vi "Facade.vi"(0 "Data In":T7, 2 "Display State In":T5, 3 "Container State":T6) -> (6 "Data Out":T7, 7 "Display State Out":T5, 8 "Action":T4)   [LabVIEW 2020, in "Input Criteria Table.xctl"]
uses:
  Input Criteria Table.xctl
  Data.vi
  Digital Input VIs/Tosca-Input Criterion.ctl
  epl-vi-lib/Utility VIs/Type Defs/Logic State.ctl
  <vilib>/_xctls/Container State.ctl
  State.vi
  <vilib>/_xctls/Action.ctl
  Input Criterion/Input Criterion.xctl
  Input Criterion/Data.vi
  <vilib>/_xctls/XControlSupport.lvlib
panel:
  in  "Crit5":T3(xcontrol)
  in  "Crit4":T3(xcontrol)
  in  "Crit3":T3(xcontrol)
  in  "Crit2":T3(xcontrol)
  in  "Crit1":T3(xcontrol)
  in  "Crit0":T3(xcontrol)
types:
  T1 = typedef "Tosca-Input Criterion.ctl" = cluster{"DigInput":i32, "State":T2, "Time (ms)":i32, "Name":string}
  T2 = typedef "Logic State.ctl" = enum16{"Low", "High", "Rising", "Falling"}
  T3 = cluster{"Criterion":T1, "Operator":i16, "visible":bool}
  T4 = typedef "XControlSupport.lvlib/Action.ctl" = cluster{"Data Changed?":bool, "State Changed?":bool, "Action Name":string}
  T5 = typedef "Input Criteria Table.xctl/State.vi" = cluster{"DI":string[], "Flags":string[]}
  T6 = typedef "XControlSupport.lvlib/Container State.ctl" = cluster{"Indicator?":bool, "Run Mode?":bool, " Refnum":refnum<vi>}
  T7 = typedef "Input Criteria Table.xctl/Data.vi" = cluster{"Name":string, "Criteria":T1[], "Operators":enum16{"AND", "OR"}[]}
  T8 = typedef "Input Criterion.xctl/Data.vi" = cluster{"Criterion":T1, "Operator":i16, "visible":bool}
  T9 = cluster{"Criteria":T1, "Operator":i32, "Visible":bool}
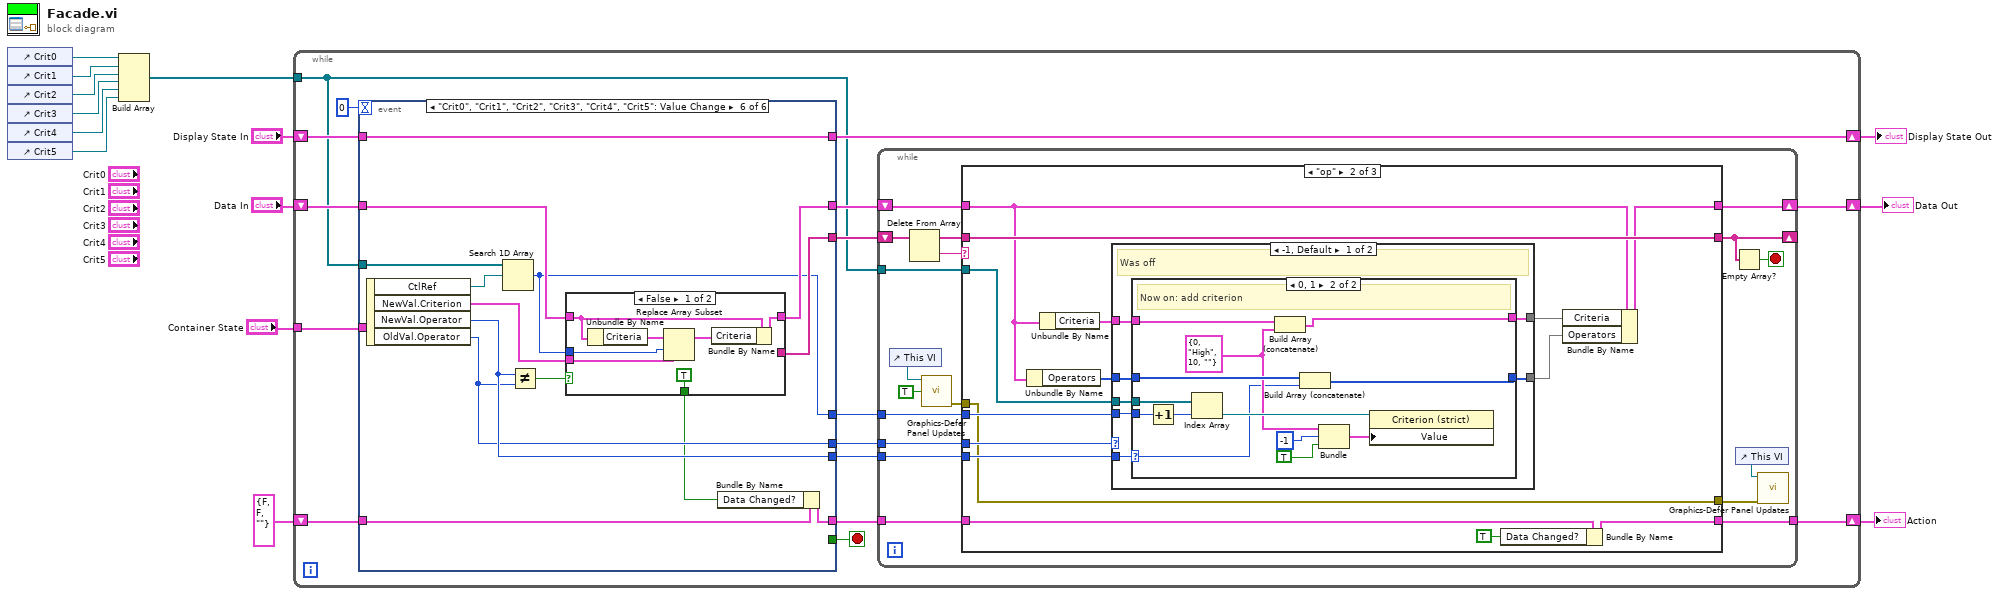
[diagram p0: block diagram]
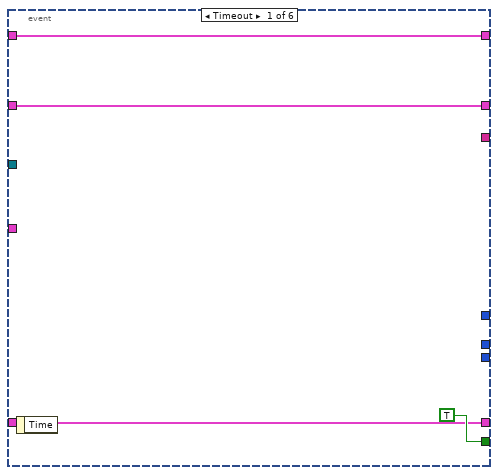
[diagram p2: hidden frame]
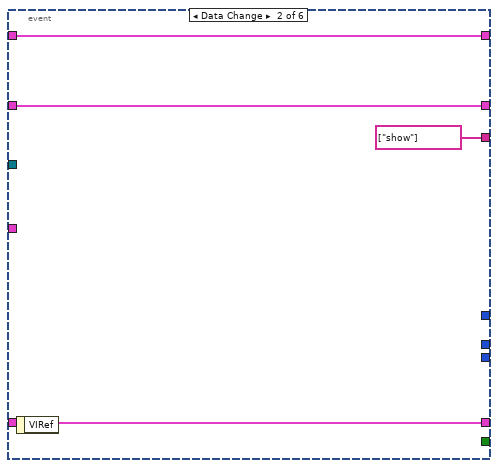
[diagram p3: hidden frame]
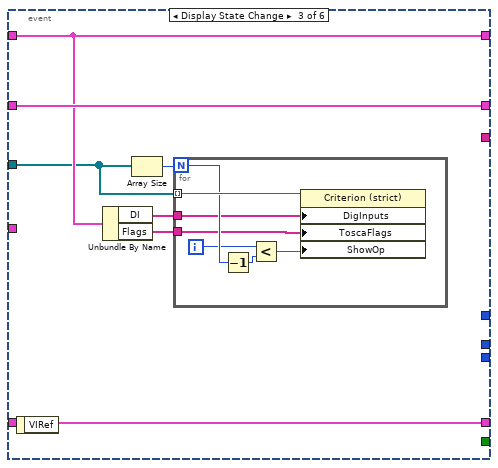
[diagram p4: hidden frame]
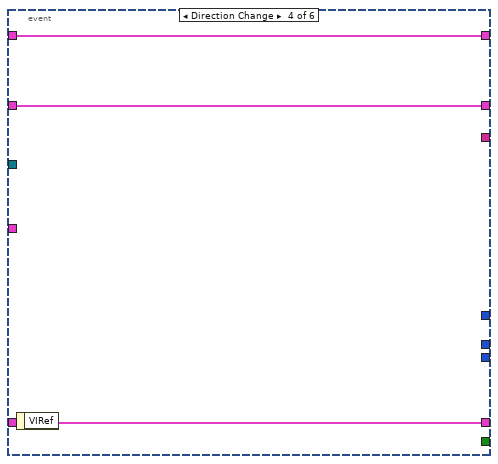
[diagram p5: hidden frame]
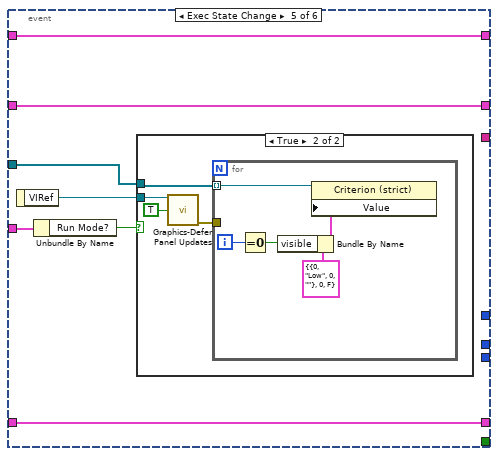
[diagram p6: hidden frame]
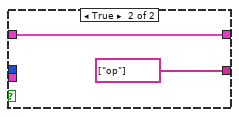
[diagram p8: hidden frame]
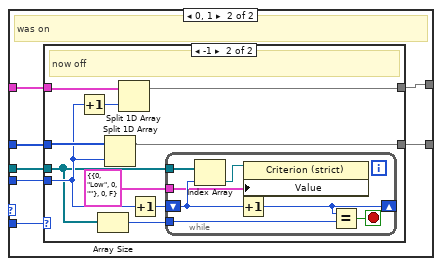
[diagram p11: hidden frame]
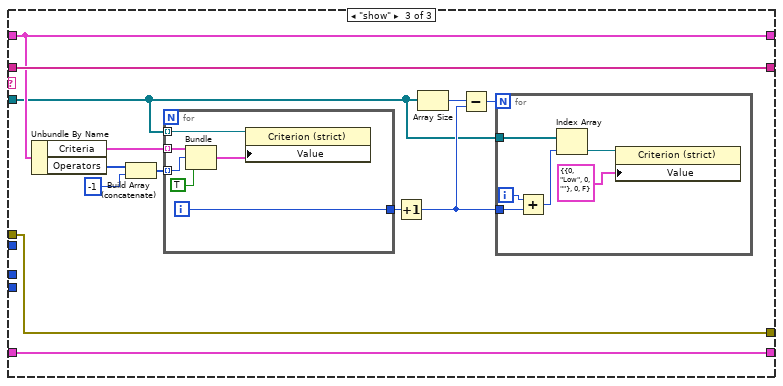
[diagram p13: hidden frame]
diagram:
  n1 = control-ref of="Crit0"() -> (w7:refnum<vi>)
  n2 = control-ref of="Crit1"() -> (w6:refnum<vi>)
  n3 = control-ref of="Crit2"() -> (w5:refnum<vi>)
  n4 = control-ref of="Crit3"() -> (w4:refnum<vi>)
  n5 = control-ref of="Crit4"() -> (w3:refnum<vi>)
  n6 = control-ref of="Crit5"() -> (w2:refnum<vi>)
  n7 = Build Array(w7, w6, w5, w4, w3, w2) -> (w1:refnum<vi>[])
  n8 = while {
    shift-right: [w29] -> w11
    shift-left: "Display State In" -> [w30]
    tunnel: "Container State" -> [w26]
    shift-right: [w18] -> w14
    shift-left: "Data In" -> [w25]
    shift-right: [w20] -> w9
    shift-left: T4 {"Data Changed?"=FALSE, "State Changed?"=FALSE, "Action Name"=""} ("Action") -> [w24]
    tunnel: w1 -> [w16]
    stop <- w28 stop-if-true
    n9 = event shown="[5] \"Crit0\", \"Crit1\", \"Crit2\", \"Crit3\", \"Crit4\", \"Crit5\": Value Change" {
      selector: _ -> [_ _ _ _ _ _]
      dyn-events: _ -> [_ _ _ _ _ _]
      timeout: 0 -> [_ _ _ _ _ _]
      tunnel: w30 -> [w32 w38 w43 w55 w62 w85]
      tunnel: [w32 w38 w43 w55 w62 w85] -> w29
      tunnel: [TRUE _ _ _ _ _] -> w28
      tunnel: w26 -> [_ _ _ _ w57 _]
      tunnel: w25 -> [w31 w36 w45 w54 w61 w77]
      tunnel: [w31 w36 w45 w54 w61 w76] -> w23
      tunnel: [w33 w37 w44 w53 w60 w75] -> w19
      tunnel: w24 -> [w33 w37 w44 w53 w60 w84]
      tunnel: w16 -> [_ _ w39 _ w58 w83]
      tunnel: [_ string[] ["show"] _ _ _ w78] -> w22
      tunnel: [_ _ _ _ _ w80] -> w21
      tunnel: [_ _ _ _ _ w73] -> w17
      tunnel: [_ _ _ _ _ w79] -> w15
      event Timeout {
        n10 = event-data() -> ()  [unwired: 1 in, 1 out]
      }
      event Data Change {
        n11 = event-data() -> ()  [unwired: 1 in, 1 out]
      }
      event Display State Change {
        n12 = event-data() -> ()  [unwired: 1 in, 1 out]
        n13 = Unbundle By Name(w43) -> ("DI"=w42:string[], "Flags"=w41:string[])
        n14 = Array Size(array=w39) -> (size(s)=w40:i32)
        n15 = for {
          N: w40 -> [w51]
          tunnel: w39 -> [w52] mode=indexing
          tunnel: w42 -> [w48]
          tunnel: w41 -> [w47]
          i -> [w49]
          n16 = Decrement(x=w51) -> (x-1=w50:i32)
          n17 = Less?(x=w49, y=w50) -> (x < y?=w46:bool)
          n18 = property class="Criterion (strict)"(reference=w52, "DigInputs"=w48, "ToscaFlags"=w47, "ShowOp"=w46) -> ()  [unwired: 1 in, 2 out]
        }
      }
      event Direction Change {
        n19 = event-data() -> ()  [unwired: 1 in, 1 out]
      }
      event Exec State Change {
        n20 = event-data() -> ("VIRef"=w59:refnum<vi>)  [unwired: 1 in]
        n21 = Unbundle By Name(w57) -> ("Run Mode?"=w56:bool)
        n22 = case shown="True" w56 {
          tunnel: w59 -> [_ w66]
          tunnel: w58 -> [_ w64]
          frame False {
          }
          frame True {
            n23 = call "Graphics-Defer Panel Updates.vi"("VI"=w66, "Defer (F)"=TRUE) -> ("error out"=w63:errorcluster)  [unwired: 12 in, 1 out]
            n24 = for {
              tunnel: w64 -> [w71] mode=indexing
              tunnel: w63 -> [_]
              i -> [w70]
              n25 = Equal To 0?(x=w70) -> (x = 0?=w69:bool)
              n26 = Bundle By Name(cluster=T8 {"Criterion"={"DigInput"=0, "State"=enum."Low", "Time (ms)"=0, "Name"=""}, "Operator"=0, "visible"=FALSE} ("Data"), "visible"=w69) -> (w68:T8)
              n27 = property class="Criterion (strict)"(reference=w71, "Value"=w68) -> ()  [unwired: 1 in, 2 out]
            }
          }
        }
      }
      event "Crit0", "Crit1", "Crit2", "Crit3", "Crit4", "Crit5": Value Change {
        n28 = event-data() -> ("CtlRef"=w82:refnum<vi>, "NewVal.Criterion"=w74:T1, "NewVal.Operator"=w80:i16, "OldVal.Operator"=w79:i16)  [unwired: 1 in]
        n29 = Search 1D Array(1D array=w83, element=w82) -> (index of element=w73:i32)  [unwired: 1 in]
        n30 = Not Equal?(x=w80, y=w79) -> (x != y?=w81:bool)
        n31 = case shown="False" w81 {
          tunnel: [_ string[] ["op"]] -> w78
          tunnel: w77 -> [w91 w93]
          tunnel: [w92 w93] -> w76
          tunnel: w74 -> [w89 _]
          tunnel: w73 -> [w87 _]
          tunnel: [TRUE _] -> w72
          frame False {
            n32 = Unbundle By Name(w91) -> ("Criteria"=w90:T1[])
            n33 = Replace Array Subset(array=w90, new element=w89, index=w87) -> (w88:T1[])
            n34 = Bundle By Name(cluster=w91, "Criteria"=w88) -> (w92:T7)
          }
          frame True {
          }
        }
        n35 = Bundle By Name(cluster=w84, "Data Changed?"=w72) -> (w75:T4)
      }
    }
    n36 = while {
      shift-right: [w109] -> _
      shift-left: w22 -> [w112]
      shift-right: [w103] -> w18
      shift-left: w23 -> [w106]
      tunnel: w21 -> [w107]
      tunnel: [w105] -> w20
      tunnel: w19 -> [w104]
      tunnel: w17 -> [w102]
      tunnel: w16 -> [w101]
      tunnel: w15 -> [w100]
      stop <- w108 stop-if-true
      n37 = control-ref of="This VI"() -> (w99:refnum<vi>)
      n38 = Delete From Array(array=w112) -> (deleted portion=w110:string, array with subset deleted=w111:string[])  [unwired: 2 in]
      n39 = call "Graphics-Defer Panel Updates.vi"("VI"=w99, "Defer (F)"=TRUE) -> ("error out"=w97:errorcluster)  [unwired: 12 in, 1 out]
      n40 = case shown="\"op\"" w110 {
        tunnel: w111 -> [w116 w131 w192]
        tunnel: [w116 w131 w192] -> w109
        tunnel: w107 -> [_ w129 _]
        tunnel: w106 -> [w114 w125 w182]
        tunnel: [w115 w120 w191] -> w105
        tunnel: w104 -> [w115 w130 w191]
        tunnel: [w114 w123 w182] -> w103
        tunnel: w102 -> [_ w126 _]
        tunnel: w101 -> [_ w128 w181]
        tunnel: w100 -> [_ w118 _]
        tunnel: w97 -> [w113 w117 w180]
        tunnel: [w113 w117 w180] -> w95
        frame "", Default {
        }
        frame "op" {
          n41 = Unbundle By Name(w125) -> ("Operators"=w127:enum16{"AND", "OR"}[])
          n42 = Unbundle By Name(w125) -> ("Criteria"=w124:T1[])
          n43 = case shown="-1, Default" w118 {
            tunnel: w128 -> [w138 w154]
            tunnel: w124 -> [w137 w159]
            tunnel: w127 -> [w136 w157]
            tunnel: w126 -> [w135 w155]
            tunnel: [w134 w160] -> w122
            tunnel: [w133 w158] -> w121
            tunnel: w129 -> [w132 w156]
            frame -1, Default {
              # "Was off"
              n44 = case shown="0, 1" w132 {
                selector: w132 -> [_ w142]
                tunnel: w138 -> [_ w149]
                tunnel: w137 -> [w140 w151]
                tunnel: w136 -> [w139 w153]
                tunnel: w135 -> [_ w148]
                tunnel: [w140 w150] -> w134
                tunnel: [w139 w152] -> w133
                frame -1, Default {
                  # "Still off: do nothing"
                }
                frame 0, 1 {
                  w145 = T1 {"DigInput"=0, "State"=enum."High", "Time (ms)"=10, "Name"=""} ("Criterion")
                  # "Now on: add criterion"
                  n45 = Increment(x=w148) -> (x+1=w147:i32)
                  n46 = Index Array(array=w149, index=w147) -> (element=w146:refnum<vi>)
                  n47 = Build Array (concatenate)(w151, w145) -> (w150:T1[])
                  n48 = Build Array (concatenate)(w153, w142) -> (w152:u16[])
                  n49 = Bundle("Criterion"=w145, i16 -1, TRUE) -> (w143:cluster{"Criterion":T1, i16, bool})  [unwired: 1 in]
                  n50 = property class="Criterion (strict)"(reference=w146, "Value"=w143) -> ()  [unwired: 1 in, 2 out]
                }
              }
            }
            frame 0, 1 {
              # "was on"
              n51 = case shown="-1" w156 {
                tunnel: [w162 w169] -> w160
                tunnel: w159 -> [w162 w170]
                tunnel: [w161 w171] -> w158
                tunnel: w157 -> [w161 w172]
                tunnel: w155 -> [_ w167]
                tunnel: w154 -> [_ w165]
                frame 0, 1, Default {
                  # "still on"
                }
                frame -1 {
                  # "now off"
                  n52 = Increment(x=w167) -> (x+1=w168:i32)
                  n53 = Array Size(array=w165) -> (size(s)=w164:i32)
                  n54 = Split 1D Array(array=w172, index=w167) -> (first subarray=w171:enum16{"AND", "OR"}[])  [unwired: 1 out]
                  n55 = Split 1D Array(array=w170, index=w168) -> (first subarray=w169:T1[])  [unwired: 1 out]
                  n56 = Increment(x=w167) -> (x+1=w166:i32)
                  n57 = while {
                    tunnel: w165 -> [w179]
                    shift-right: [w175] -> _
                    shift-left: w166 -> [w177]
                    tunnel: w164 -> [w174]
                    tunnel: T8 {"Criterion"={"DigInput"=0, "State"=enum."Low", "Time (ms)"=0, "Name"=""}, "Operator"=0, "visible"=FALSE} ("Data") -> [w173]
                    stop <- w176 stop-if-true
                    n58 = Index Array(array=w179, index=w177) -> (element=w178:refnum<vi>)
                    n59 = Increment(x=w177) -> (x+1=w175:i32)
                    n60 = property class="Criterion (strict)"(reference=w178, "Value"=w173) -> ()  [unwired: 1 in, 2 out]
                    n61 = Equal?(x=w175, y=w174) -> (x = y?=w176:bool)
                  }
                }
              }
            }
          }
          n62 = Bundle By Name(cluster=w130, "Data Changed?"=TRUE) -> (w120:T4)
          n63 = Bundle By Name(cluster=w125, "Criteria"=w122, "Operators"=w121) -> (w123:T7)
        }
        frame "show" {
          n64 = Unbundle By Name(w182) -> ("Criteria"=w183:T1[], "Operators"=w184:enum16{"AND", "OR"}[])
          n65 = Build Array (concatenate)(w184, -1) -> (w186:i32[])
          n66 = for {
            tunnel: w183 -> [w197] mode=indexing
            tunnel: w181 -> [w198] mode=indexing
            tunnel: w186 -> [w196] mode=indexing
            tunnel: [w194] -> w187
            i -> [w194]
            n67 = Bundle("Criteria"=w197, "Operator"=w196, "Visible"=TRUE) -> (w195:T9)  [unwired: 1 in]
            n68 = property class="Criterion (strict)"(reference=w198, "Value"=w195) -> ()  [unwired: 1 in, 2 out]
          }
          n69 = Increment(x=w187) -> (x+1=w190:i32)
          n70 = Array Size(array=w181) -> (size(s)=w188:i32)
          n71 = Subtract(x=w188, y=w190) -> (x-y=w189:i32)
          n72 = for {
            N: w189 -> [_]
            tunnel: w190 -> [w203]
            tunnel: w181 -> [w204]
            i -> [w202]
            n73 = Add(x=w202, y=w203) -> (x+y=w201:i32)
            n74 = Index Array(array=w204, index=w201) -> (element=w200:refnum<vi>)
            n75 = property class="Criterion (strict)"(reference=w200, "Value"=T8 {"Criterion"={"DigInput"=0, "State"=enum."Low", "Time (ms)"=0, "Name"=""}, "Operator"=0, "visible"=FALSE} ("Data")) -> ()  [unwired: 1 in, 2 out]
          }
        }
      }
      n76 = Empty Array?(array=w109) -> (empty?=w108:bool)
      n77 = control-ref of="This VI"() -> (w96:refnum<vi>)
      n78 = call "Graphics-Defer Panel Updates.vi"("VI"=w96, "error in (no error)"=w95) -> ()  [unwired: 12 in, 2 out]
    }
  }
  "Display State Out" <- w11
  "Data Out" <- w14
  "Action" <- w9
